vi "Marker Or Cursor A B And Table.vi"(4 "o/x Marker Value (0,0)":dbl min=-9.99999e+37 max=9.99999e+37 format="%^.3e", 6 "o And x Marker(0:oMarkerVal)":u32(ring) items=["o Marker Value", "x Marker value", "Store Sweep Sange", "Partial Sweep Range On", "Partial Sweep Range Off", "o Marker Max A", "o Marker Min A", "o Marker Max B", "o Marker Min B", "Store Analysys Range", "Partial Analysis Range On", "Partial Analysis Range Off"], 7 "Marker/Line Curs(1:o Marker On)":u32(ring)=1 items=["Marker And Line Cursor Off", "o Marker On", "o Marker And x Marker On"], 8 "error in (no error)":errorcluster, 9 "o Marker Value (0,0)":dbl min=-9.99999e+37 max=9.99999e+37 format="%^.3e", 10 "o Marker (0:o Marker Value)":u32(ring) items=["o Marker Value", "o Marker Max of A", "o Marker Min of A", "o Marker Max of B", "o Marker Min of B"], 11 "VISA resource name":refnum<visa-resource-name>) -> (0 "error out":errorcluster, 3 "VISA resource name out":refnum<visa-resource-name>)   [LabVIEW 2010, in "Agilent 4194.lvlib"]
doc: "This function supports marker and cursor operations for mode A - B and Table.\n\nNotes:\n\n(1) o is a sign for the first type of cursor/marker.\n\n(2) x is a sign for the second type of cursor/marker."
uses:
  <instrlib>/Agilent 4194/Agilent 4194.lvlib
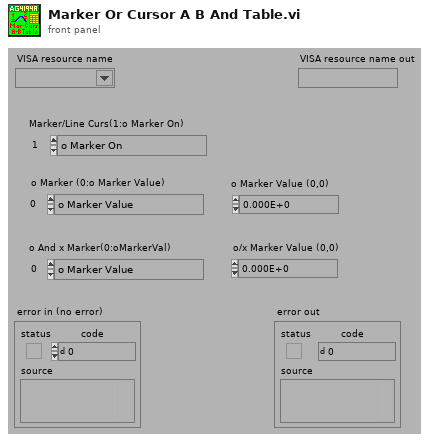
[diagram p1: front panel]
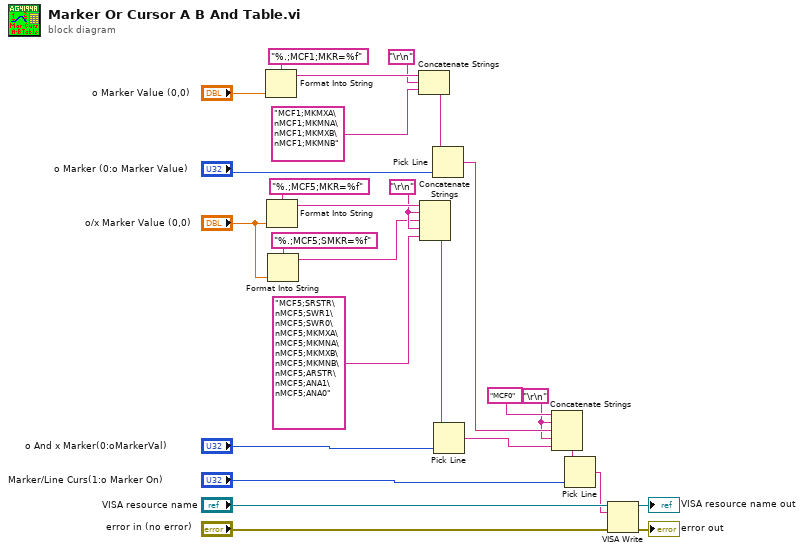
[diagram p0: block diagram]
diagram:
  w1 = "\r\n"
  w18 = "\r\n"
  n1 = Format Into String(format string="%.;MCF1;MKR=%f", "o Marker Value (0,0)") -> (resulting string=w26:string)  [unwired: 2 in, 1 out]
  n2 = Format Into String(format string="%.;MCF5;MKR=%f", "o/x Marker Value (0,0)") -> (resulting string=w21:string)  [unwired: 2 in, 1 out]
  n3 = Format Into String(format string="%.;MCF5;SMKR=%f", "o/x Marker Value (0,0)") -> (resulting string=w17:string)  [unwired: 2 in, 1 out]
  n4 = Concatenate Strings(w26, "\r\n", "MCF1;MKMXA\nMCF1;MKMNA\nMCF1;MKMXB\nMCF1;MKMNB") -> (w23:string)
  n5 = Concatenate Strings(w21, w18, w17, w18, "MCF5;SRSTR\nMCF5;SWR1\nMCF5;SWR0\nMCF5;MKMXA\nMCF5;MKMNA\nMCF5;MKMXB\nMCF5;MKMNB\nMCF5;ARSTR\nMCF5;ANA1\nMCF5;ANA0") -> (w20:string)
  n6 = Pick Line(multi-line string=w23, line index="o Marker (0:o Marker Value)") -> (output string=w15:string)  [unwired: 1 in]
  n7 = Pick Line(multi-line string=w20, line index="o And x Marker(0:oMarkerVal)") -> (output string=w5:string)  [unwired: 1 in]
  n8 = Concatenate Strings("MCF0", w1, w15, w1, w5) -> (w4:string)
  n9 = Pick Line(multi-line string=w4, line index="Marker/Line Curs(1:o Marker On)") -> (output string=w3:string)  [unwired: 1 in]
  n10 = VISA Write(VISA resource name="VISA resource name", write buffer=w3, error in (no error)="error in (no error)") -> (VISA resource name out=→"VISA resource name out":refnum<visa-resource-name>, error out=→"error out":errorcluster)  [unwired: 1 out]
